vi "FilterRepeating.vi"(9 "Error in":errorcluster) -> (1 "Error out":errorcluster, 2 "Repeating error filtered?":bool)   [LabVIEW 2017, in "GPError.lvlib"]
doc: "Clears the error(s) and/or warning(s) on <B>Error in</B> if <B>Error in</B> is identical with the last time this VI was called. This is useful to guard some function from spamming an error handler repeatedly with the same error over and over, if you expect the errant function to recover again later and can live with only a single passing of the repeating error.\n\nTo maintain the filter the error on <B>Error in</B> must be the same at every call, so if this VI is called repeatedly with two alternating errors for instance, they will both be able to get through thus defeating the repeat-filter.\n\nThis function considers two errors equal only if their code, status, source and description fields are all identical. Two errors that differ only in timestamp are considered equal as well however.\n\nThis VI supports filtering appended errors, in which case the entire appended error collection must be identical with the last run for the filter to activate.\n\nThis VI is inlined.\n\nSteen Schmidt\nGPower\n11/7 2013"
uses:
  GPError.lvlib
panel:
  # "Copyright © 2011-2013\nSteen Schmidt, GPower\nSee enclosed license file for terms and conditions"
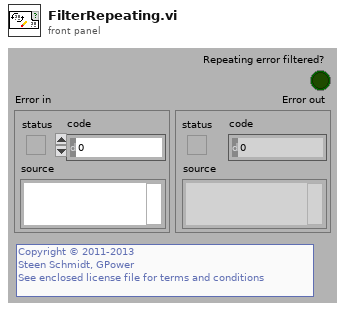
[diagram p1: front panel]
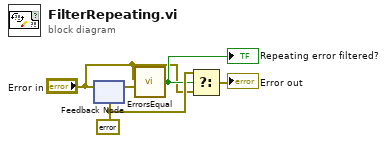
[diagram p0: block diagram]
diagram:
  w4 = errorcluster {"status"=FALSE, "code"=0, "source"=""} ("error out")
  n1 = feedback-in #1("Error in") -> ()
  n2 = feedback #1(w4) -> (w3:errorcluster)
  n3 = call "ErrorsEqual.vi"("Error in 2"=w3, "Error in 1"="Error in") -> ("Errors equal?"=w2:bool)  [unwired: 4 in]
  "Repeating error filtered?" <- w2
  n4 = Select(t=w4, s=w2, f="Error in") -> (s? t:f=→"Error out":errorcluster)
